vi "niFGEN - 3 Sessions Unregistered.vi"(8 "error in":errorcluster) -> (0 "error out":errorcluster, 3 "data out":T1)   [LabVIEW 2020, in "MeasurementServerTests.lvlib"]
uses:
  MeasurementServerTests.lvlib
  Runtime/MeasurementLink Session Management/Session Reservation/Data.ctl
  Runtime/MeasurementLink Session Management/Session Reservation/Session and Driver Info.ctl
  Runtime/MeasurementLink Session Management Client/RPC Messages/ni_measurementlink_sessionmanagement_v1_SessionInformation.ctl
  Runtime/MeasurementLink Session Management Client/RPC Messages/nidevice_grpc_Session.ctl
  Runtime/MeasurementLink Session Management Client/RPC Messages/ni_measurementlink_sessionmanagement_v1_ChannelMapping.ctl
  54c6e20d-b9da-4053-bdae-38eddc7e8fbe.vi
  <vilib>/JDP Science/JSONtext/JSON text to Variant.vi
  <vilib>/JDP Science/JSONtext/LVClass Serializer/JSONtext LVClass Serializer.lvclass
  Runtime/MeasurementLink Session Management Client/MeasurementLink Session Management Client.lvlib
  Runtime/MeasurementLink Session Management/Session Reservation/Session Reservation.lvclass
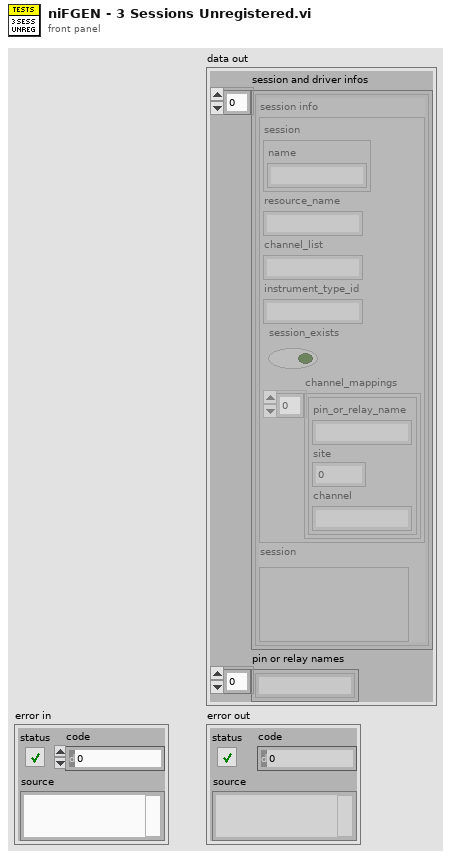
[diagram p1: front panel]
types:
  T1 = typedef "MeasurementLink Session Management.lvlib/Session Reservation.lvclass/Data.ctl" = cluster{"session and driver infos":T2[], "pin or relay names":string[]}
  T2 = typedef "MeasurementLink Session Management.lvlib/Session Reservation.lvclass/Session and Driver Info.ctl" = cluster{"session info":T3, "session":variant}
  T3 = typedef "MeasurementLink Session Management Client.lvlib/ni_measurementlink_sessionmanagement_v1_SessionInformation.ctl" = cluster{"session":T4, "resource_name":string, "channel_list":string, "instrument_type_id":string, "session_exists":bool, "channel_mappings":T5[]}
  T4 = typedef "MeasurementLink Session Management Client.lvlib/nidevice_grpc_Session.ctl" = cluster{"name":string}
  T5 = typedef "MeasurementLink Session Management Client.lvlib/ni_measurementlink_sessionmanagement_v1_ChannelMapping.ctl" = cluster{"pin_or_relay_name":string, "site":i32, "channel":string}
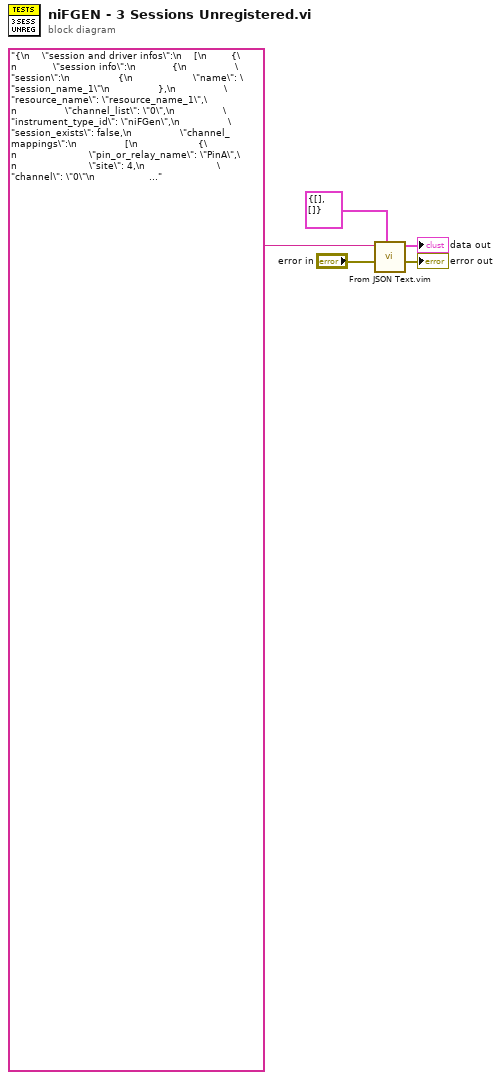
[diagram p0: block diagram]
diagram:
  n1 = call "From JSON Text.vim"("Data Type and Default Value"=T1 {"session and driver infos"=[], "pin or relay names"=[]} ("data"), "error in (no error)"="error in", "JSON"="{\n    \"session and driver infos\":\n    [\n        {\n            \"session info\":\n            {\n                \"session\":\n                {\n                    \"name\": \"session_name_1\"\n                },\n                \"resource_name\": \"resource_name_1\",\n                \"channel_list\": \"0\",\n                \"instrument_type_id\": \"niFGen\",\n                \"session_exists\": false,\n                \"channel_mappings\":\n                [\n                    {\n                        \"pin_or_relay_name\": \"PinA\",\n                        \"site\": 4,\n                        \"channel\": \"0\"\n                    }\n                ]\n            }\n        },\n        {\n            \"session info\":\n            {\n                \"session\":\n                {\n                    \"name\": \"session_name_2\"\n                },\n                \"resource_name\": \"resource_name_2\",\n                \"channel_list\": \"0\",\n                \"instrument_type_id\": \"niFGen\",\n                \"session_exists\": false,\n                \"channel_mappings\":\n                [\n                    {\n                        \"pin_or_relay_name\": \"PinB\",\n                        \"site\": 4,\n                        \"channel\": \"0\"\n                    }\n                ]\n            }\n        },\n        {\n            \"session info\":\n            {\n                \"session\":\n                {\n                    \"name\": \"session_name_3\"\n                },\n                \"resource_name\": \"resource_name_3\",\n                \"channel_list\": \"0\",\n                \"instrument_type_id\": \"niFGen\",\n                \"session_exists\": false,\n                \"channel_mappings\":\n                [\n                    {\n                        \"pin_or_relay_name\": \"PinC\",\n                        \"site\": 4,\n                        \"channel\": \"0\"\n                    }\n                ]\n            }\n        },\n    ]\n}") -> ("error out"=→"error out":errorcluster, "Data out"=→"data out":T1)  [unwired: 7 in]
